vi "Read Roles.vi"(8 "error in (no error)":errorcluster, 11 "KickoffAllyPlayVSS in":refnum<class "KickoffAllyPlayVSS.lvclass">) -> (0 "error out":errorcluster, 2 "Roles":T1, 3 "KickoffAllyPlayVSS out":refnum<class "KickoffAllyPlayVSS.lvclass">)   [LabVIEW 2020, in "KickoffAllyPlayVSS.lvclass"]
uses:
  KickoffAllyPlayVSS.lvclass
  NormalAttackerRoleVSS_class/NormalAttackerRoleVSS.lvclass
  KeeperRoleVSS_class/KeeperRoleVSS.lvclass
  DefenderAreaRoleVSS_class/DefenderAreaRoleVSS.lvclass
  KickoffAllyPlayVSS.lvclass/KickoffAllyPlayVSS.ctl
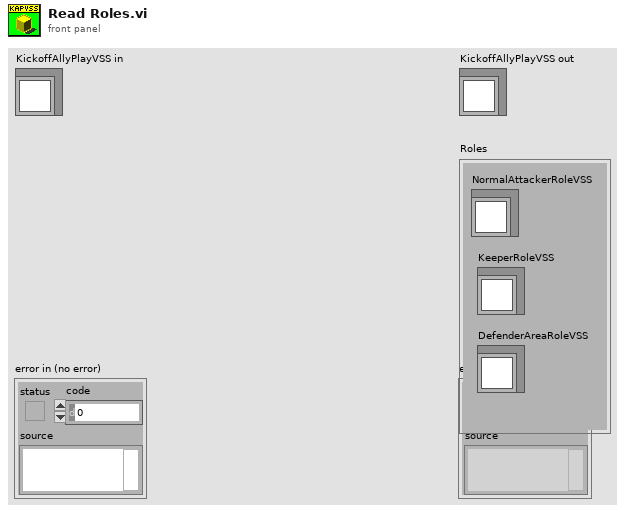
[diagram p1: front panel]
types:
  T1 = cluster{"NormalAttackerRoleVSS":refnum<class "NormalAttackerRoleVSS.lvclass">, "KeeperRoleVSS":refnum<class "KeeperRoleVSS.lvclass">, "DefenderAreaRoleVSS":refnum<class "DefenderAreaRoleVSS.lvclass">}
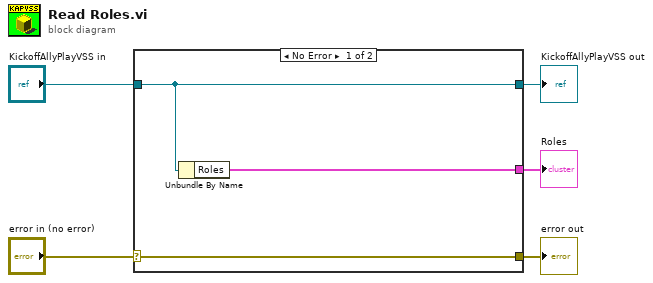
[diagram p0: block diagram]
diagram:
  n1 = case shown="No Error" "error in (no error)" {
    selector: "error in (no error)" -> [w8 w9]
    tunnel: [w8 w9] -> w4
    tunnel: [w7 w10] -> w2
    tunnel: "KickoffAllyPlayVSS in" -> [w7 w10]
    tunnel: [w6 _] -> w1
    frame No Error {
      n2 = Unbundle By Name(w7) -> ("Roles"=w6:T1)
    }
    frame Error {
    }
  }
  "error out" <- w4
  "KickoffAllyPlayVSS out" <- w2
  "Roles" <- w1
